vi "transition.vi"(8 "error in (no error)":errorcluster, 10 "ContextData In":refnum<class "ContextData.lvclass">, 11 "Exit in":refnum<class "Exit.lvclass">) -> (0 "error out":errorcluster, 2 "ContextData Out":refnum<class "ContextData.lvclass">, 3 "Exit out":refnum<class "State.lvclass">)   [LabVIEW 2019, in "Exit.lvclass"]
uses:
  Exit.lvclass
  C:/Users/Felipe-PC/Documents/Projetos/Projetos Github/OOP-State-Machine/State/State.lvclass
  State/State.lvclass
  ContextData/ContextData.lvclass
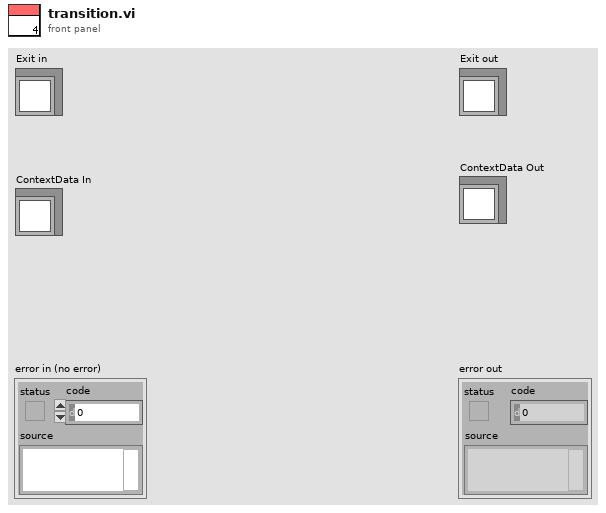
[diagram p1: front panel]
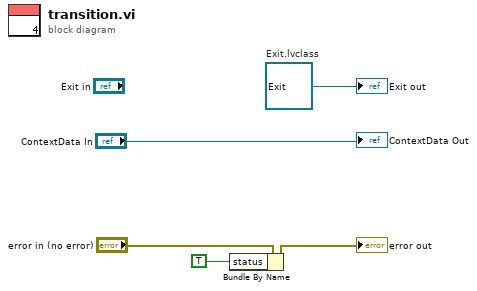
[diagram p0: block diagram]
diagram:
  w1 = refnum<class "Exit.lvclass"> refnum  # Exit.lvclass
  n1 = Bundle By Name(cluster="error in (no error)", "status"=TRUE) -> (→"error out":errorcluster)
  "Exit out" <- w1
  "ContextData Out" <- "ContextData In"
